vi "RPStoSpeed.vi"(10 "RPS":dbl) -> (2 "Speed":dbl)   [LabVIEW 2012]
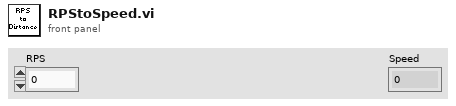
[diagram p1: front panel]
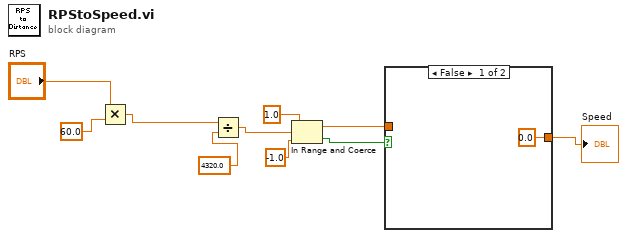
[diagram p0: block diagram]
diagram:
  n1 = Multiply(x="RPS", y=60.0) -> (x*y=w7:dbl)
  n2 = Divide(x=w7, y=4320.0) -> (x/y=w4:dbl)
  n3 = In Range and Coerce(upper limit=1.0, x=w4, lower limit=-1.0) -> (coerced(x)=w2:dbl, In Range?=w3:bool)
  n4 = case shown="False" w3 {
    tunnel: w2 -> [_ w12]
    tunnel: [0.0 ("upper limit") w12] -> w1
    frame False {
    }
    frame True {
    }
  }
  "Speed" <- w1
